vi "BundleItem.vi"(1 "Value":string, 2 "Key":string) -> (0 "Item":T1)   [LabVIEW 2014, in "Raspberry Pi Compatible Compiler for LabVIEW.lvlib" / "PythonConfiguration.lvclass"]
uses:
  PythonConfiguration.lvclass
  TypeDefs/ItemTD.ctl
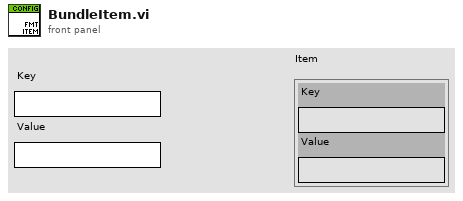
[diagram p1: front panel]
types:
  T1 = typedef "Raspberry Pi Compatible Compiler for LabVIEW.lvlib/PythonConfiguration.lvclass/ItemTD.ctl" = cluster{"Key":string, "Value":string}
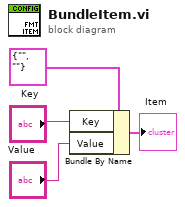
[diagram p0: block diagram]
diagram:
  n1 = Bundle By Name(cluster=T1 {"Key"="", "Value"=""} ("Item"), "Key"="Key", "Value"="Value") -> (→"Item":T1)
